vi "test.vi"() -> ()   [LabVIEW 2020]
uses:
  <vilib>/Utility/file.llb/Read Delimited Spreadsheet (DBL).vi
panel:
  out "크기 2":i32
  out "혼합된 신호 그래프 2":cluster{"all rows":dbl[], "all rows":dbl[]}[](graph)
  out "크기":i32
  out "Heading_T":dbl
  out "TM_Y(long)":dbl format="%-#_10g M"
  out "TM_X(lat)":dbl format="%-#_10g M"
  in  "?":enum32{"State", "ETC"}(tab)
  in  "stop":bool
  in  "file path (dialog if empty)":path caption="RDDF"
  out "XY Graph 2":T1(graph)
  in  "Refresh":bool
  in  "A/M":bool=TRUE
  in  "Serial Name":refnum<visa-resource-name>="COM8"
  out "ERP_Serial_DATA(RAW)":string
  in  "Vel":dbl=4.0 format="%#_13g"
  out "Index(near vehicle)":i32
  out "WP_no.":i32
  out "x_lat_path":dbl[](array[numeric])
  out "y_long_path":dbl[](array[numeric])
  out "vel. path":dbl[](array[numeric])
  out "Path_Vel_arr":dbl[](array[numeric])
  out "Path_long_arr":dbl[](array[numeric])
  out "Path_lat_arr":dbl[](array[numeric])
  out "ERP_Receive":T2
  out "Steer_CMD(Deg)":dbl
  out "CMD_2_ERP":T3
  out "Brake":u8
  in  "Number of Points":i32=200
  in  "Magnitude":dbl
  in  "X Origin":dbl
  in  "Y Origin":dbl
  out "XY Graph":cluster{dbl[], dbl[]}(graph)
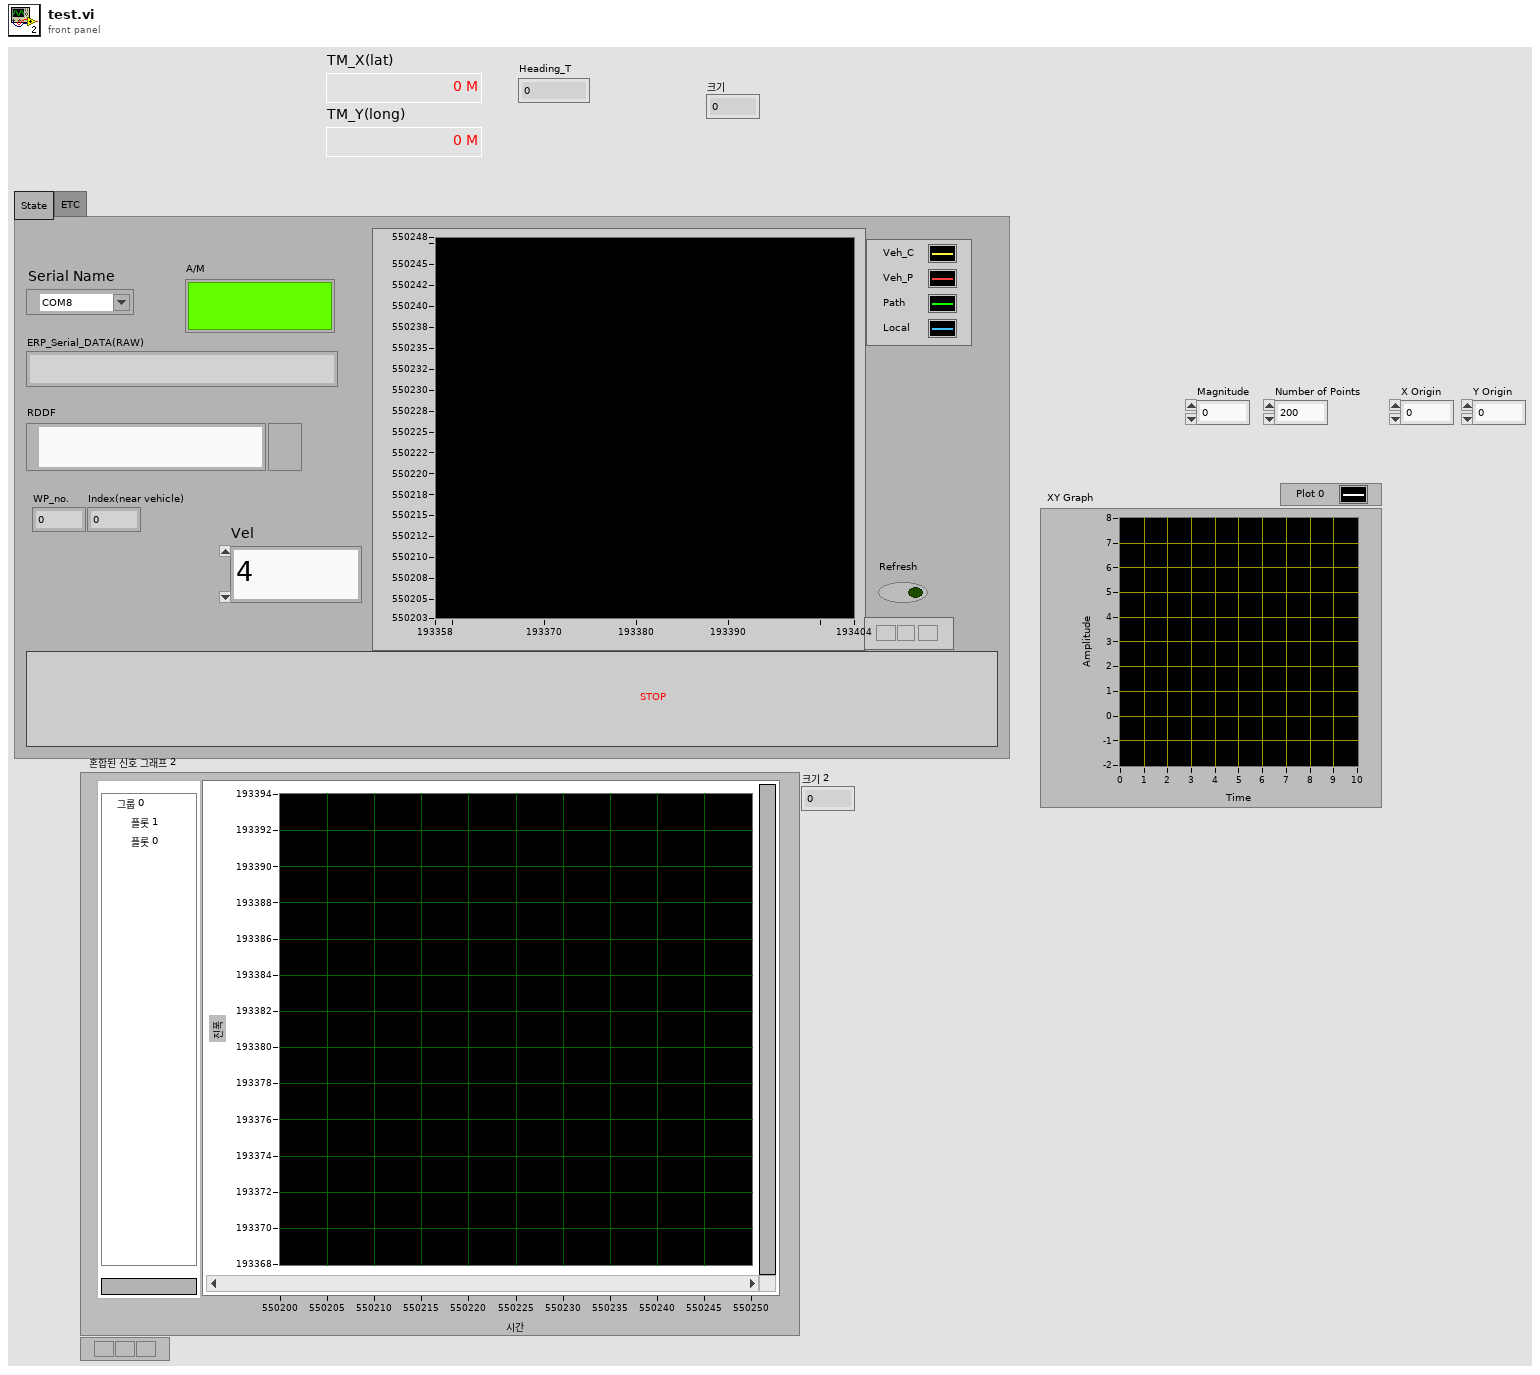
[diagram p1: front panel]
types:
  T1 = cluster{"y_long_path":dbl[], "x_lat_path":dbl[]}[]
  T2 = cluster{"AorM":u8, "E-Stop":u8, "F_B":u8, "Speed":u16, "Steer":i16, "Brake":u8, "Encoder":u8, "Encoder 2":u8, "Encoder 3":u8, "Encoder 4":u8, "ALIVE":u8, "ETX_0":u8, "ETX_0 2":u8}
  T3 = cluster{"F/B":u8, "Speed":u16, "Steer":i16, "A/M":u8, "Brake":u8}
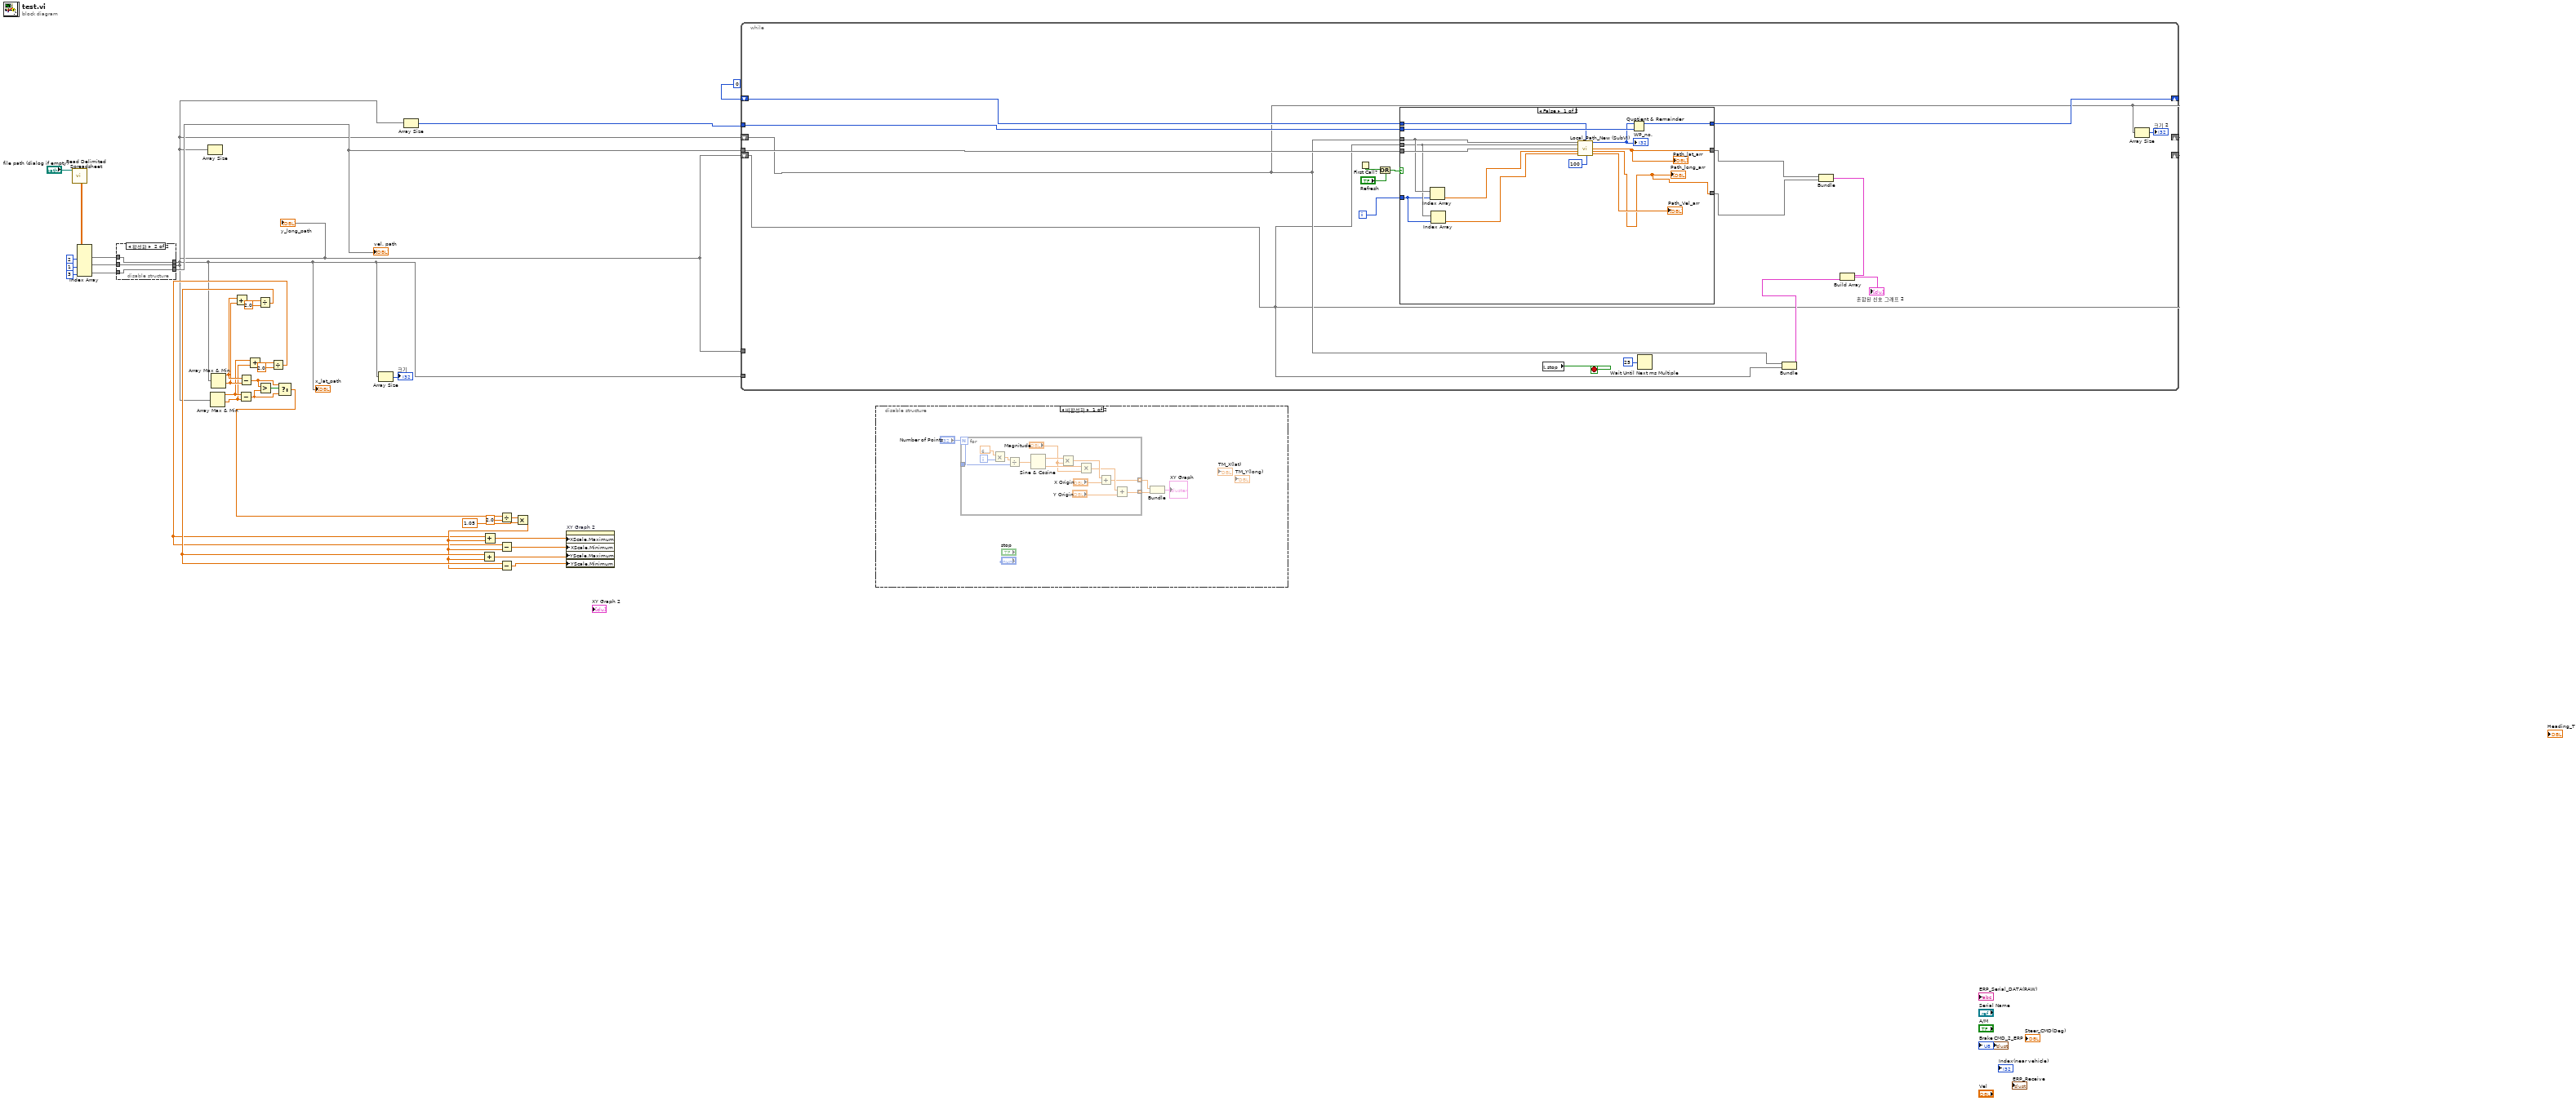
[diagram p0: block diagram]
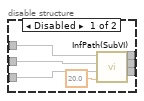
[diagram p3: hidden frame]
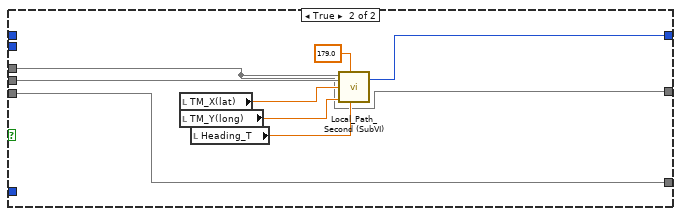
[diagram p4: hidden frame]
diagram:
  n1 = call-poly <vilib>:"Read Delimited Spreadsheet.vi"("file path (dialog if empty)"="file path (dialog if empty)") -> ("all rows"=w7:dbl[][])  [unwired: 9 in, 5 out]
  n2 = Index Array(array=w7, index (col) #1=2 ("비활성화된 인덱스 (열)"), index (col) #2=1 ("인덱스 (열)"), index (col) #3=3 ("인덱스 (열)")) -> (element #1=w33:dbl[], element #2=w32:dbl[], element #3=w31:dbl[])  [unwired: 3 in]
  n3 = disable-structure shown="활성화" {
    disable-tunnel: w33 -> [w43 w46]
    disable-tunnel: w32 -> [w42 w45]
    disable-tunnel: w31 -> [w41 w44]
    disable-tunnel: [w40 w45] -> w2
    disable-tunnel: [w39 w44] -> w8
    disable-tunnel: [w38 w46] -> w1
    frame Disabled {
      n4 = call "InfPath(SubVI).vi"("Mod dist."=20.0, "vel."=w41, "y_long"=w42, "x_lat"=w43) -> ("vel. path"=w39:dbl[], "y_long_path"=w40:dbl[], "x_lat_path"=w38:dbl[])  [unwired: 1 out]
    }
    frame Enabled {
    }
  }
  "x_lat_path" <- w1
  "y_long_path" <- w2
  "vel. path" <- w8
  n5 = Array Size(array=w1) -> ()  [unwired: 1 out]
  n6 = Array Max & Min(array=w2) -> (max value=w19:dbl, min value=w18:dbl)  [unwired: 2 out]
  n7 = Array Max & Min(array=w1) -> (max value=w25:dbl, min value=w24:dbl)  [unwired: 2 out]
  n8 = Add(x=w25, y=w24) -> (x+y=w22:dbl)
  n9 = Subtract(x=w19, y=w18) -> (x-y=w28:dbl)
  n10 = Subtract(x=w25, y=w24) -> (x-y=w29:dbl)
  n11 = Add(x=w19, y=w18) -> (x+y=w21:dbl)
  n12 = Divide(x=w22, y=2.0) -> (x/y=w15:dbl)
  n13 = Greater?(x=w29, y=w28) -> (0:w30:bool)
  n14 = Divide(x=w21, y=2.0) -> (x/y=w5:dbl)
  n15 = Select(t=w29, s=w30, f=w28) -> (s? t:f=w26:dbl)
  n16 = Array Size(array=w1) -> (size(s)=→"크기":i32)
  n17 = Array Size(array=w1) -> (size(s)=w9:i32)
  n18 = Divide(x=w26, y=2.0) -> (x/y=w17:dbl)
  n19 = Multiply(x=w17, y=1.05) -> (x*y=w14:dbl)
  n20 = Add(x=w15, y=w14) -> (x+y=w12:dbl)
  n21 = Add(x=w5, y=w14) -> (x+y=w10:dbl)
  n22 = Subtract(x=w5, y=w14) -> (x-y=w11:dbl)
  n23 = Subtract(x=w15, y=w14) -> (x-y=w13:dbl)
  n24 = property on="XY Graph 2" class="XYGraph (엄격한)"("XScale.Maximum"=w10, "XScale.Minimum"=w11, "YScale.Maximum"=w12, "YScale.Minimum"=w13) -> ()  [unwired: 2 in, 2 out]
  n25 = while {
    tunnel: w8 -> [w63]
    tunnel: w9 -> [w62]
    shift-right: [w61] -> _
    shift-left: 0 ("Index0") -> [w50]
    tunnel: w1 -> [_]
    tunnel: w2 -> [_]
    shift-right: [w48] -> _
    shift-left: w1 -> [w48]
    shift-right: [w47] -> _
    shift-left: w2 -> [w47]
    i -> [w49]
    stop <- w64 stop-if-true
    n26 = First Call?() -> (First Call?: T/F=w59:bool)
    n27 = Or(x=w59, y="Refresh") -> (x .or. y?=w60:bool)
    n28 = case shown="False" w60 {
      tunnel: w48 -> [w72 w80]
      tunnel: w47 -> [w71 w86]
      tunnel: w50 -> [w75 _]
      tunnel: w63 -> [w73 w79]
      tunnel: w62 -> [w77 _]
      tunnel: [w78 w81] -> w61
      tunnel: [w66 w80] -> w52
      tunnel: [w65 w79] -> w53
      tunnel: w49 -> [w70 _]
      frame False {
        n29 = Index Array(array=w72, index=w70) -> (element=w69:dbl)
        n30 = Index Array(array=w71, index=w70) -> (element=w68:dbl)
        n31 = call "Local_Path_New (SubVI).vi"("x_lat_arr"=w72, "WP no_pre"=w75, "y_long_arr"=w71, "vel_arr"=w73, "x_lat_c"=w69, "y_long_c"=w68, "# of pnt"=100) -> ("INDEX(Near Point)"=w67:i32, "Lat(Local)"=w66:dbl[], "Long(Local)"=w65:dbl[], "Vel(Local)"=→"Path_Vel_arr":dbl[])  [unwired: 5 in]
        "Path_lat_arr" <- w66
        "Path_long_arr" <- w65
        "WP_no." <- w67
        n32 = Quotient & Remainder(x=w67, y=w77) -> (x-y*floor(x/y)=w78:i32)  [unwired: 1 out]
      }
      frame True {
        n33 = local read "TM_X(lat)"() -> (w85:dbl)
        n34 = local read "TM_Y(long)"() -> (w84:dbl)
        n35 = local read "Heading_T"() -> (w83:dbl)
        n36 = call "Local_Path_Second (SubVI).vi"("heading_deg"=w83, "heading_limit"=179.0, "y_long"=w84, "x_lat"=w85, "Y_long_path"=w86, "X_lat_path"=w80) -> ("Index(near vehicle)"=w81:i32)  [unwired: 1 out]
      }
    }
    n37 = local read "stop"() -> (w64:bool)
    n38 = Wait Until Next ms Multiple(millisecond multiple=u32 25) -> ()  [unwired: 1 out]
    n39 = Bundle("all rows"=w48, "all rows"=w47) -> (w54:cluster{"all rows":dbl[], "all rows":dbl[]})  [unwired: 1 in]
    n40 = Bundle("all rows"=w52, "all rows"=w53) -> (w56:cluster{"all rows":dbl[], "all rows":dbl[]})  [unwired: 1 in]
    n41 = Build Array(w56, w54) -> (→"혼합된 신호 그래프 2":cluster{"all rows":dbl[], "all rows":dbl[]}[])
    n42 = Array Size(array=w48) -> (size(s)=→"크기 2":i32)
  }
  n43 = disable-structure shown="비활성화" {
    frame Disabled {
      n44 = for {
        N: "Number of Points" -> [_]
        tunnel: "Number of Points" -> [w102]
        tunnel: [w92] -> w87 mode=indexing
        tunnel: [w91] -> w88 mode=indexing
        i -> [w104]
        n45 = Multiply(x=6.283185307179586, y=w104) -> (x*y=w103:dbl)
        n46 = Divide(x=w103, y=w102) -> (x/y=w100:dbl)
        n47 = Sine & Cosine(0:w100) -> (1:w99:dbl, 2:w98:dbl)
        n48 = Multiply(x=w99, y="Magnitude") -> (x*y=w96:dbl)
        n49 = Multiply(x=w98, y="Magnitude") -> (x*y=w95:dbl)
        n50 = Add(x=w96, y="X Origin") -> (x+y=w92:dbl)
        n51 = Add(x=w95, y="Y Origin") -> (x+y=w91:dbl)
      }
      n52 = Bundle(w87, w88) -> (→"XY Graph":cluster{dbl[], dbl[]})  [unwired: 1 in]
    }
    frame Enabled {
    }
  }
